vi "VII Slave Read Bytes.vi"(6 "pLen":u16, 7 "pReadData":string, 8 "error in (no error)":errorcluster, 9 "I2CIndex":i32, 10 "DevIndex":i32, 11 "DevType":i32) -> (0 "error out":errorcluster, 3 "function return":i32, 4 "pLen out":u16, 5 "pReadData out":string)   [LabVIEW 2011, in "ControlI2C.lvlib"]
doc: "int __stdcall VII_SlaveReadBytes(int DevType,int DevIndex,int I2CIndex,unsigned char* pReadData,unsigned short *pLen);"
uses:
  ControlI2C.lvlib
  1234/Ginkgo_Driver.dll
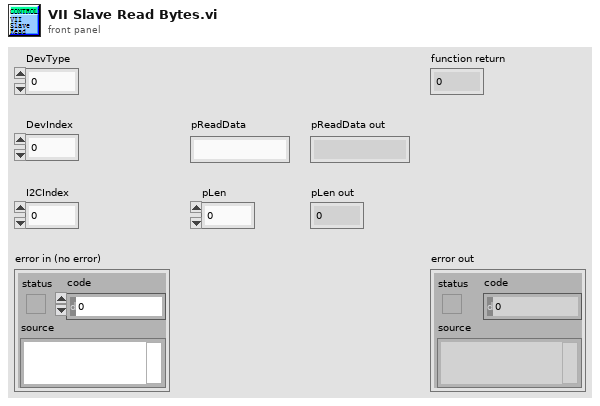
[diagram p1: front panel]
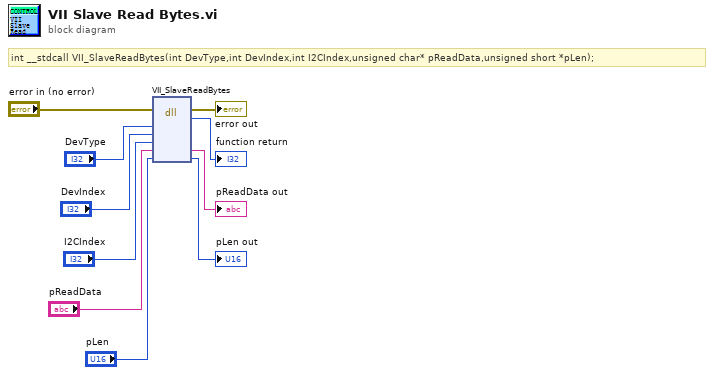
[diagram p0: block diagram]
diagram:
  # "int __stdcall VII_SlaveReadBytes(int DevType,int DevIndex,int I2CIndex,unsigned char* pReadData,unsigned short *pLen);"
  n1 = dll-call lib="E:/Project/vt_ginkgo/truck/Ginkgo Driver/vs2010/Ginkgo_USB-I2C&SPI&CAN_API_v2.0.3.3/lib/labview_32bit/1234/Ginkgo_Driver.*" fn="VII_SlaveReadBytes"(error in="error in (no error)", "DevType"="DevType", "DevIndex"="DevIndex", "I2CIndex"="I2CIndex", "pReadData"="pReadData", "pLen"="pLen") -> (error out=→"error out":errorcluster, →"function return":i32, "pReadData"=→"pReadData out":string, "pLen"=→"pLen out":u16)  [unwired: 5 in, 1 out]
